vi "QR code reader test.vi"() -> ()   [LabVIEW 2021, in "Test VIs.lvclass"]
uses:
  Test VIs/Test VIs.lvclass
  Classes/Controller/Camera/QR Code Reader/QR Code Reader.lvclass
  C:/Users/HEP/Documents/GitHub/Gantry/UCSB-Gantry-HEP-main/Classes/Controller/Camera/Camera.lvclass
  Classes/Controller/Camera/Camera.lvclass
panel:
  out "Image":T1(plugin-control)
  in  "Stop":bool
  out "QR Code Reader.lvclass":refnum<class "QR Code Reader.lvclass">
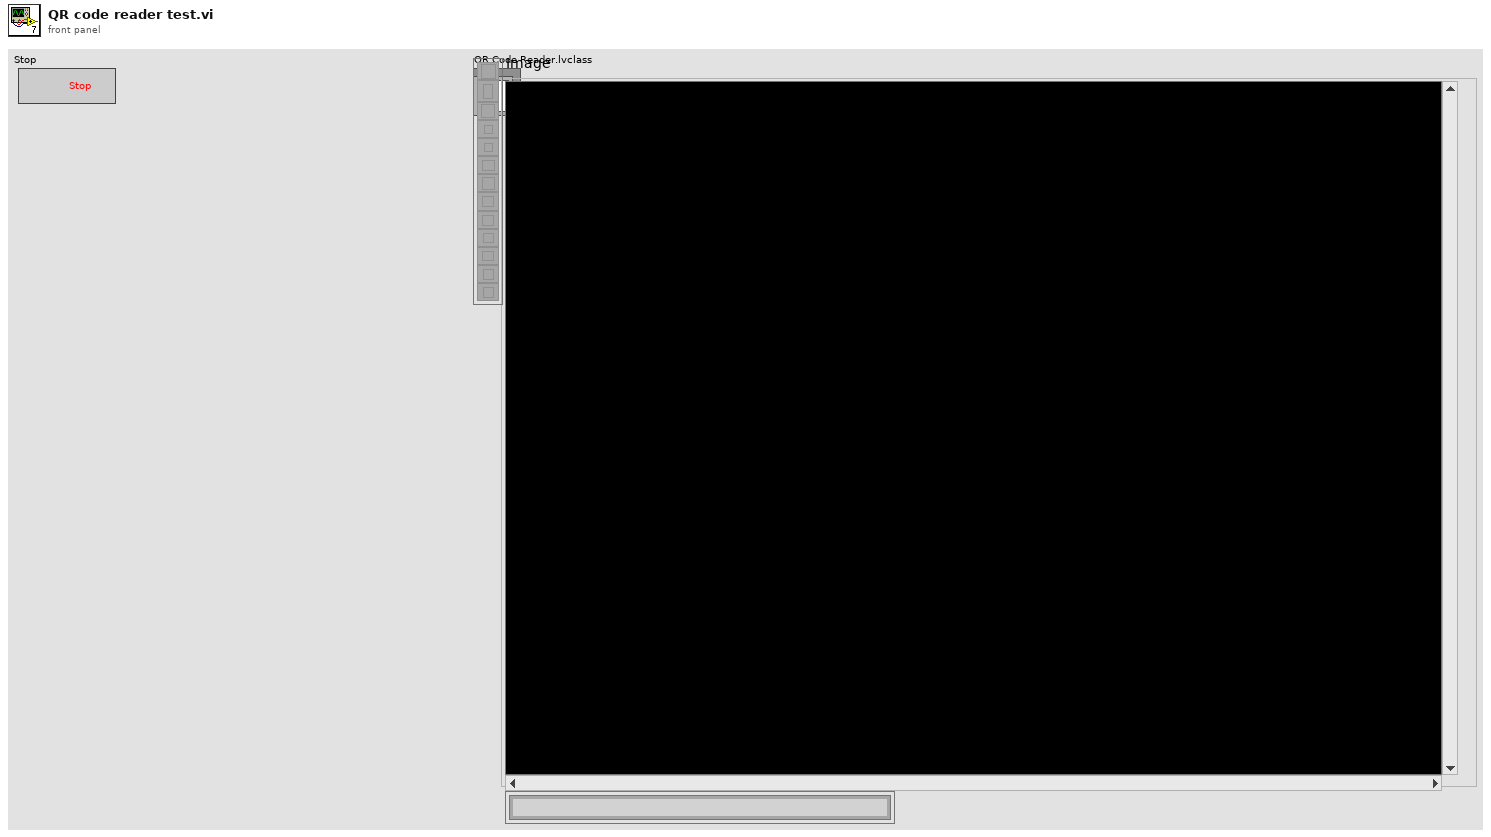
[diagram p1: front panel]
types:
  T1 = typedef "IMAQ Image.ctl" = refnum<image>
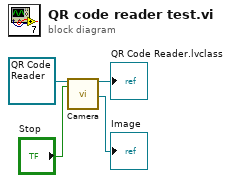
[diagram p0: block diagram]
diagram:
  n1 = call "Camera.vi"("Camera in"=refnum<class "QR Code Reader.lvclass"> refnum ("QR Code Reader.lvclass"), "Stop"="Stop") -> ("Camera out"=→"QR Code Reader.lvclass":refnum<class "QR Code Reader.lvclass">, "Image"=→"Image":T1)  [unwired: 10 in, 6 out]
